vi "DisignPattern.vi"() -> ()   [LabVIEW 2018]
panel:
  in  "정지 2":bool
  out "배열":bool[](array[boolean])
  out "상태":T1(ring)
  out "배출 상품명 2":string
  out "웰치스 LED 2":bool
  out "콜라 LED 2":bool
  out "환타 LED 2":bool
  out "사이다 LED 2":bool
  out "현재 잔액 2":dbl
  in  "정지":bool
  in  "거스름돈 반환":bool
  out "배출 상품명":string
  out "현재 잔액":dbl
  out "웰치스 LED":bool
  in  "웰치스":bool
  out "콜라 LED":bool
  in  "콜라":bool
  out "환타 LED":bool
  in  "환타":bool
  in  "1000원":bool
  in  "500원":bool
  in  "100원":bool
  out "사이다 LED":bool
  in  "사이다":bool
  in  "50원":bool
  in  "10원":bool
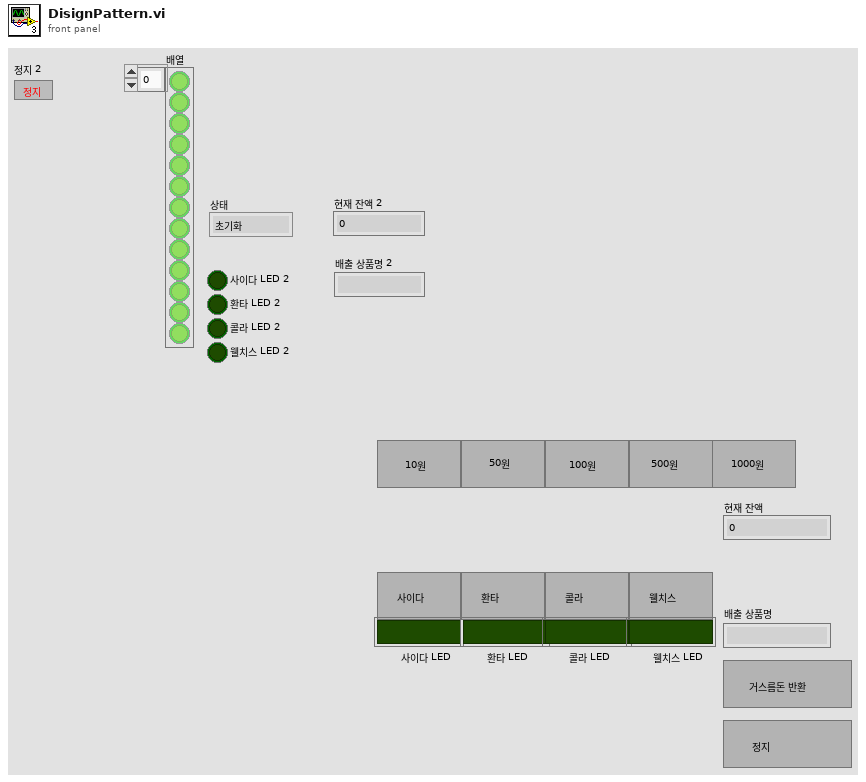
[diagram p1: front panel]
types:
  T1 = enum16{"초기화", "대기", "10원", "50원", "100원", "500원", "1000원", "디스플레이 업데이트", "사이다", "콜라", "환타", "웰치스", "거스름돈 반환", "종료"}
  T2 = cluster{"현재 잔액":dbl, "사이다 LED":bool, "환타 LED":bool, "콜라 LED":bool, "웰치스 LED":bool, "배출 상품명":string, "상태":enum16{"초기화", "대기", "10원", "50원", "100원", "500원", "1000원", "디스플레이 업데이트", "사이다", "콜라", "환타", "웰치스", "거스름돈 반환", "종료"}}
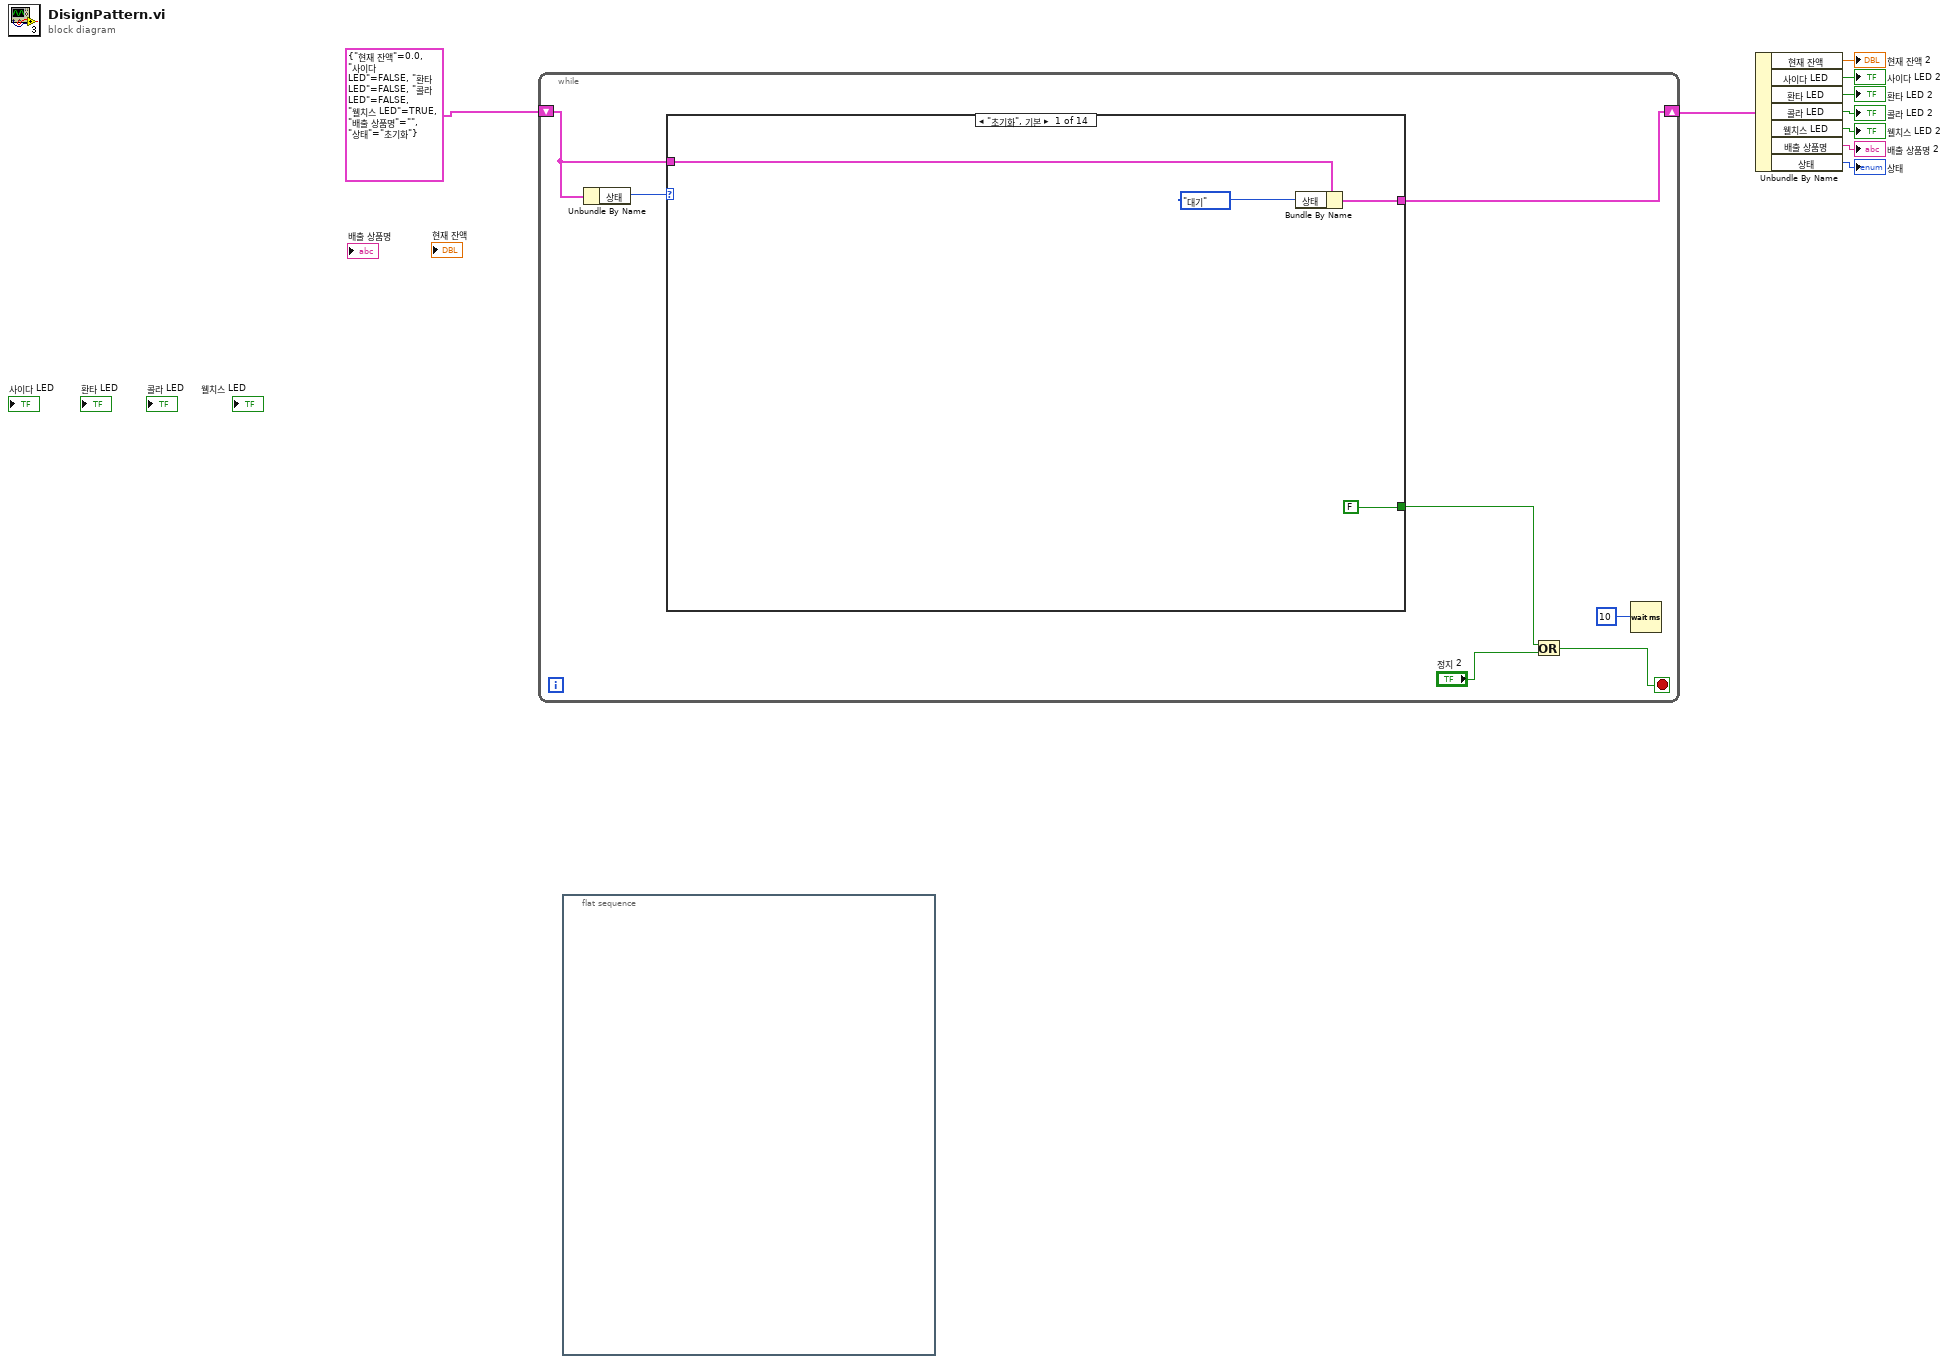
[diagram p0: block diagram]
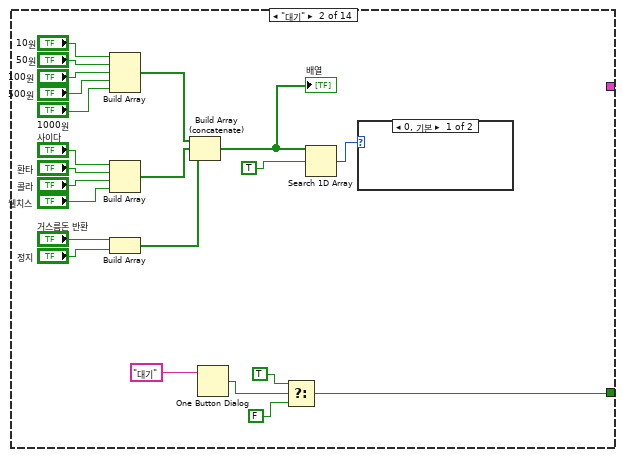
[diagram p2: hidden frame]
diagram:
  n1 = while {
    shift-right: [w14] -> w8
    shift-left: T2 {"현재 잔액"=0.0, "사이다 LED"=FALSE, "환타 LED"=FALSE, "콜라 LED"=FALSE, "웰치스 LED"=TRUE, "배출 상품명"="", "상태"=enum."초기화"} -> [w15]
    stop <- w10 stop-if-true
    n2 = Unbundle By Name(w15) -> ("상태"=w16:T1)
    n3 = case shown="\"초기화\", 기본" w16 {
      tunnel: w15 -> [w20 _ _ _ _ _ _ _ _ _ _ _ _ _]
      tunnel: [w18 _ _ _ _ _ _ _ _ _ _ _ _ _] -> w14
      tunnel: [FALSE w21 _ _ _ _ _ _ _ _ _ _ _ _] -> w11
      frame "초기화", Default {
        n4 = Bundle By Name(cluster=w20, "상태"=T1."대기") -> (w18:T2)
      }
      frame "대기" {
        n5 = Build Array("10원", "50원", "100원", "500원", "1000원") -> (w31:bool[])
        n6 = Build Array("사이다", "환타", "콜라", "웰치스") -> (w30:bool[])
        n7 = Build Array("거스름돈 반환", "정지") -> (w29:bool[])
        n8 = Build Array (concatenate)(w31, w30, w29) -> (w26:bool[])
        "배열" <- w26
        n9 = One Button Dialog(message="대기") -> (true=w24:bool)  [unwired: 1 in]
        n10 = Select(t=TRUE, s=w24, f=FALSE) -> (s? t:f=w21:bool)
        n11 = Search 1D Array(1D array=w26, element=TRUE) -> (index of element=w27:i32)  [unwired: 1 in]
        n12 = case shown="0, 기본" w27 {
          frame 0, Default {
          }
          frame 1 {
          }
        }
      }
      frame "10원" {
      }
      frame "50원" {
      }
      frame "100원" {
      }
      frame "500원" {
      }
      frame "1000원" {
      }
      frame "디스플레이 업데이트" {
      }
      frame "사이다" {
      }
      frame "콜라" {
      }
      frame "환타" {
      }
      frame "웰치스" {
      }
      frame "거스름돈 반환" {
      }
      frame "종료" {
      }
    }
    n13 = Or(x=w11, y="정지 2") -> (x .or. y?=w10:bool)
    n14 = Wait (ms)(milliseconds to wait=10) -> ()  [unwired: 1 out]
  }
  n15 = flat-sequence {
    frame #0 {
    }
  }
  n16 = Unbundle By Name(w8) -> ("현재 잔액"=→"현재 잔액 2":dbl, "사이다 LED"=→"사이다 LED 2":bool, "환타 LED"=→"환타 LED 2":bool, "콜라 LED"=→"콜라 LED 2":bool, "웰치스 LED"=→"웰치스 LED 2":bool, "배출 상품명"=→"배출 상품명 2":string, "상태"=→"상태":T1)
